vi "OrientationCCW2(L).vi"() -> (0 "Array of Operations (out)":T1[](array[typedef])=[{"Device"=enum."Servo", "Angles"=[enum."0°", enum."-90°", enum."0°"], "Grips"=[], "NoWaits"=[FALSE, FALSE, FALSE]}, {"Device"=enum."Grip", "Angles"=[], "Grips"=[TRUE, FALSE, TRUE], "NoWaits"=[FALSE, FALSE, FALSE]}, {"Device"=enum."Servo", "Angles"=[enum."0°", enum."0°", enum."0°"], "Grips"=[], "NoWaits"=[FALSE, FALSE, FALSE]}, {"Device"=enum."Grip", "Angles"=[], "Grips"=[FALSE, TRUE, TRUE], "NoWaits"=[FALSE, FALSE, FALSE]}, {"Device"=enum."Servo", "Angles"=[enum."-90°", enum."0°", enum."0°"], "Grips"=[], "NoWaits"=[FALSE, FALSE, FALSE]}, {"Device"=enum."Grip", "Angles"=[], "Grips"=[TRUE, TRUE, FALSE], "NoWaits"=[FALSE, FALSE, FALSE]}, {"Device"=enum."Servo", "Angles"=[enum."-90°", enum."0°", enum."+90°"], "Grips"=[], "NoWaits"=[FALSE, FALSE, FALSE]}, {"Device"=enum."Grip", "Angles"=[], "Grips"=[TRUE, FALSE, TRUE], "NoWaits"=[FALSE, FALSE, FALSE]}, {"Device"=enum."Servo", "Angles"=[enum."0°", enum."0°", enum."0°"], "Grips"=[], "NoWaits"=[FALSE, FALSE, FALSE]}, {"Device"=enum."Servo", "Angles"=[enum."0°", enum."-90°", enum."0°"], "Grips"=[], "NoWaits"=[FALSE, FALSE, FALSE]}, {"Device"=enum."Grip", "Angles"=[], "Grips"=[TRUE, TRUE, TRUE], "NoWaits"=[FALSE, FALSE, FALSE]}])   [LabVIEW 2017]
uses:
  Projekt-RubikLibrary/RubikOps.ctl
  Projekt-RubikLibrary/ServoAbsAngleControl.ctl
  Projekt-RubikLibrary/RubikLibrary.lvlib
panel:
  in  "Array of Operations":T1[](array[typedef])=[{"Device"=enum."Servo", "Angles"=[enum."0°", enum."-90°", enum."0°"], "Grips"=[], "NoWaits"=[FALSE, FALSE, FALSE]}, {"Device"=enum."Grip", "Angles"=[], "Grips"=[TRUE, FALSE, TRUE], "NoWaits"=[FALSE, FALSE, FALSE]}, {"Device"=enum."Servo", "Angles"=[enum."0°", enum."0°", enum."0°"], "Grips"=[], "NoWaits"=[FALSE, FALSE, FALSE]}, {"Device"=enum."Grip", "Angles"=[], "Grips"=[FALSE, TRUE, TRUE], "NoWaits"=[FALSE, FALSE, FALSE]}, {"Device"=enum."Servo", "Angles"=[enum."+90°", enum."0°", enum."0°"], "Grips"=[], "NoWaits"=[FALSE, FALSE, FALSE]}, {"Device"=enum."Grip", "Angles"=[], "Grips"=[TRUE, TRUE, FALSE], "NoWaits"=[FALSE, FALSE, FALSE]}, {"Device"=enum."Servo", "Angles"=[enum."+90°", enum."0°", enum."-90°"], "Grips"=[], "NoWaits"=[FALSE, FALSE, FALSE]}, {"Device"=enum."Grip", "Angles"=[], "Grips"=[TRUE, FALSE, TRUE], "NoWaits"=[FALSE, FALSE, FALSE]}, {"Device"=enum."Servo", "Angles"=[enum."0°", enum."0°", enum."0°"], "Grips"=[], "NoWaits"=[FALSE, FALSE, FALSE]}, {"Device"=enum."Grip", "Angles"=[enum."0°", enum."-90°", enum."0°"], "Grips"=[FALSE, TRUE, TRUE], "NoWaits"=[FALSE, FALSE, FALSE]}, {"Device"=enum."Servo", "Angles"=[enum."+90°", enum."0°", enum."0°"], "Grips"=[FALSE, FALSE, TRUE], "NoWaits"=[FALSE, FALSE, FALSE]}, {"Device"=enum."Grip", "Angles"=[enum."0°", enum."-90°", enum."0°"], "Grips"=[TRUE, TRUE], "NoWaits"=[FALSE, FALSE, FALSE]}, {"Device"=enum."Servo", "Angles"=[enum."+90°", enum."0°", enum."-90°"], "Grips"=[], "NoWaits"=[FALSE, FALSE, FALSE]}, {"Device"=enum."Grip", "Angles"=[enum."0°", enum."-90°", enum."0°"], "Grips"=[TRUE, FALSE, TRUE], "NoWaits"=[FALSE, FALSE, FALSE]}, {"Device"=enum."Servo", "Angles"=[enum."0°", enum."0°", enum."0°"], "Grips"=[], "NoWaits"=[FALSE, FALSE, FALSE]}, {"Device"=enum."Servo", "Angles"=[enum."0°", enum."-90°", enum."0°"], "Grips"=[], "NoWaits"=[FALSE, FALSE, FALSE]}, {"Device"=enum."Grip", "Angles"=[enum."0°", enum."-90°", enum."0°"], "Grips"=[TRUE, TRUE, TRUE], "NoWaits"=[FALSE, FALSE, FALSE]}]
  # "Rotate Rubik's Cube"
  # "Turn Cube clockwise (view from left servo or\ngreen face).\nUse in Orientation FSM.\nCompare to OrientationCCW(L).vi"
  # "OrientationCW(L).vi"
  # "This is the first turn of the cube"
  # "This is the second  turn of the cube"
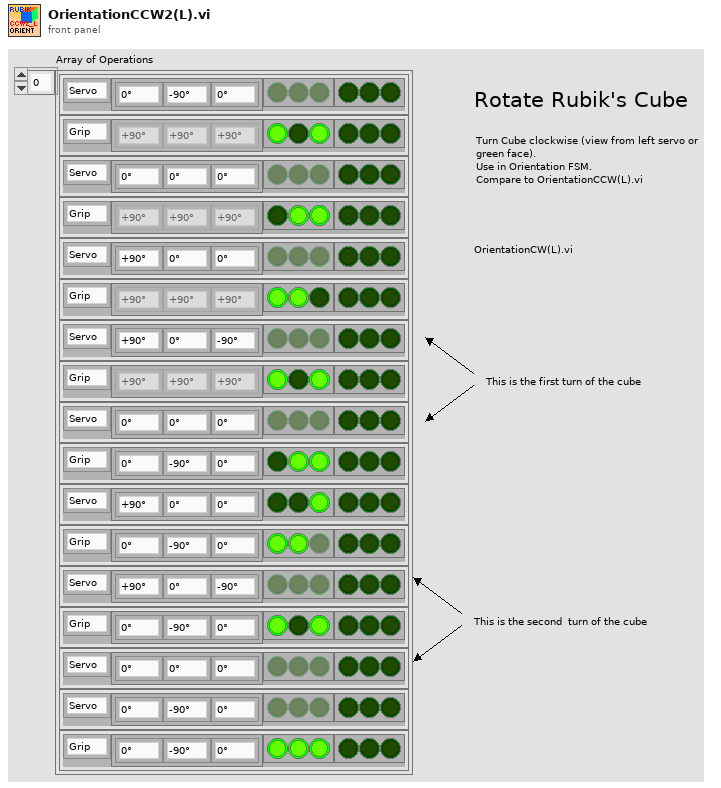
[diagram p1: front panel]
types:
  T1 = typedef "RubikLibrary.lvlib/RubikOps.ctl" = cluster{"Device":enum16{"Servo", "Grip"}, "Angles":T2[], "Grips":bool[], "NoWaits":bool[]}
  T2 = typedef "RubikLibrary.lvlib/ServoAbsAngleControl.ctl" = enum16{"+90°", "0°", "-90°"}
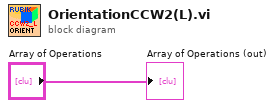
[diagram p0: block diagram]
diagram:
  "Array of Operations (out)" <- "Array of Operations"
